vi "Connect.vi"(8 "error in":errorcluster, 11 "36234A in":refnum<class "36234A.lvclass">) -> (0 "error out":errorcluster, 3 "36234A out":refnum<class "36234A.lvclass">)   [LabVIEW 2019, in "36234A.lvlib" / "36234A.lvclass"]
doc: "This disconnect routine is a must override from the Instrument Class\nChildren Classes are responsible for handling the override, but the parent class is an intermediary and must contain the override functions to maintain the rules for the method."
uses:
  Library/36234A.lvclass
  C:/Users/Public/Documents/Development/builds/Instruments/Instruments.lvlibp/Library/Instruments.lvclass
  Library/36234A.lvclass/36234A.ctl
  builds/Instruments/Instruments.lvlibp/Accessors/Read Resource.vi
  builds/Instruments/PowerSupply.lvlibp/Library/PowerSupply.lvclass
  <instrlib>/Keysight E36000 Series/Keysight E36000 Series.lvlib
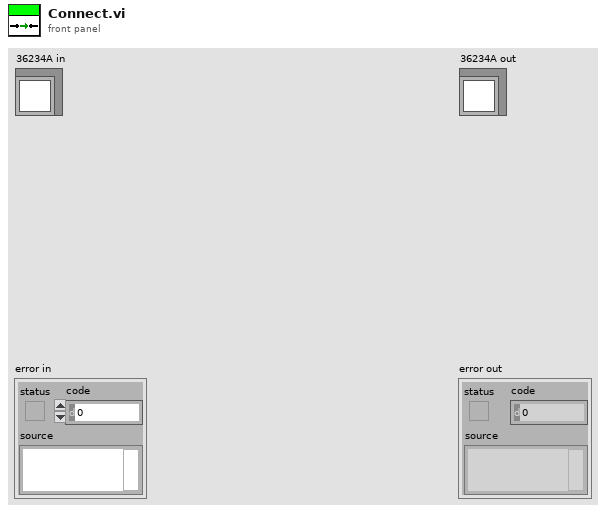
[diagram p1: front panel]
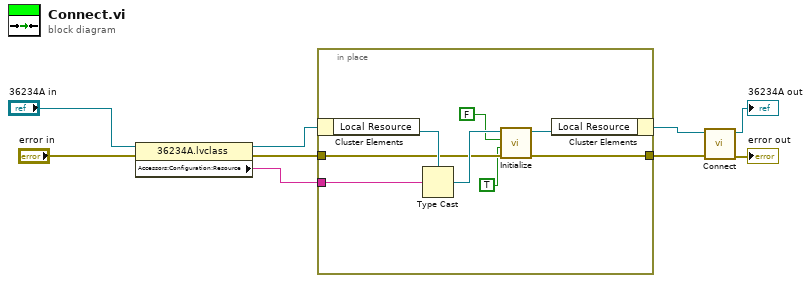
[diagram p0: block diagram]
diagram:
  n1 = property class="36234A.lvclass"(reference="36234A in", error in="error in") -> (reference out=w5:refnum<class "36234A.lvclass">, error out=w4:errorcluster, "Accessors:Configuration:Resource"=w3:string)
  n2 = in-place {
    in-place-border: w4 -> [w13]
    in-place-border: w3 -> [w16]
    in-place-border: [w12] -> w1
    n3 = in-place-cluster #1(w5) -> ("Local Resource"=w17:refnum<visa-resource-name>)
    n4 = Type Cast(type=w17, x=w16) -> (*(type *) &x=w15:refnum<visa-resource-name>)
    n5 = call <instrlib>:"Initialize.vi"("error in (no error)"=w13, "Reset (True)"=TRUE, "ID Query (True)"=FALSE, "VISA resource name"=w15) -> ("error out"=w12:errorcluster, "VISA resource name out"=w14:refnum<visa-resource-name>)  [unwired: 6 in]
    n6 = in-place-cluster #1("Local Resource"=w14) -> (w2:refnum<class "36234A.lvclass">)
  }
  n7 = call-parent "Connect.vi"("error in"=w1, "PowerSupply in"=w2) -> ("error out"=→"error out":errorcluster, "PowerSupply out"=→"36234A out":refnum<class "36234A.lvclass">)  [unwired: 8 in]
